vi "Update GUI - Waveform Chart.vi"(6 "Timestamp (optional)":timestamp, 8 "error in (no error)":errorcluster, 9 "Point value":dbl, 10 "GUI Item Name":string, 11 "uService Template in":refnum<class "Father of all uServices.lvclass">) -> (0 "error out":errorcluster, 3 "uService Template out":refnum<class "Father of all uServices.lvclass">)   [LabVIEW 2026, in "TALOS.lvlib" / "Father of all uServices.lvlib" / "Father of all uServices.lvclass"]
doc: "This VI adds a point to the selected Waveform Chart. If not provided externally, this VI will use the time of calling as the timestamp for the point given. \nNote: to properly work, the corresponding indicator in the uService GUI needs to be connected to an empty waveform chart in the Block Diagram of the uService GUI."
uses:
  Father of all uServices.lvclass
  Father of all uServices.lvclass/Father of all uServices.ctl
  Ancestor/Ancestor/Ancestor.lvclass/Ancestor.ctl
  Support VIs/Substitute Error.vi
  Support VIs/Generate Error.vi
  FGV/Error Memory/Get Error Description.vi
  Support VIs/Get PC name.vi
  Ancestor/Ancestor/Read ID.vi
  Support VIs/Get Class Name.vi
  <vilib>/Utility/error.llb/Clear Errors.vi
  FGV/Error Memory/Error Memory Core.vi
  <vilib>/AdvancedString/Delimited String to 1D String Array.vi
  <vilib>/AdvancedString/Delimited String to 1D String Array (string).vi
  Support VIs/Circus Root Path.vi
  FGV/Error Memory/Error Crt Lvl checker.vi
  FGV/Error Memory/Error Memory Core.vi/40c8088d-b597-4017-91af-faa98e00292e.vi
  FGV/Error Memory/Error Memory Core.vi/d4a3ab98-063c-4e44-b43d-fbdcfe6c2be2.vi
  Support VIs/Global Memory.vi
  <vilib>/Utility/LVClass/Get LV Class Name.vi
  Support VIs/Is in Packed Library.vi
  Support VIs/TALOS Root path.vi
  Support VIs/Read CSV worksheet.vi
  Support VIs/Global Constants.vi
  <vilib>/Utility/error.llb/General Error Handler.vi
  Support VIs/Error Log.vi
  Ancestor/Ancestor/Ancestor.lvclass
  <vilib>/Comparison/Equal/Equal Functor/Equal Functor.lvclass
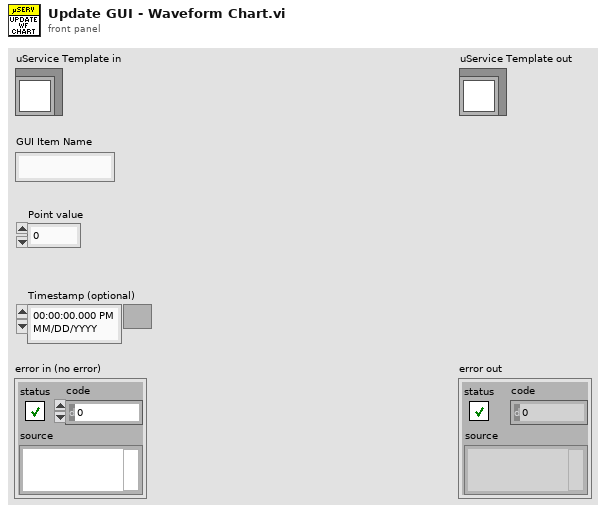
[diagram p1: front panel]
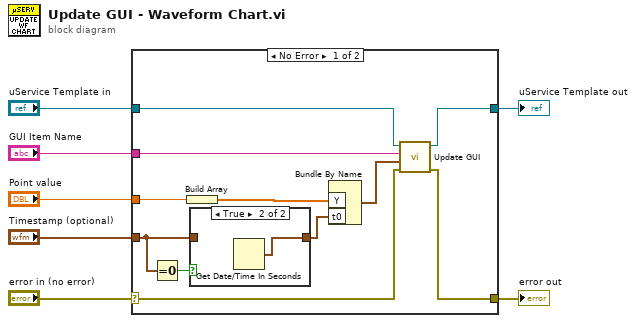
[diagram p0: block diagram]
diagram:
  n1 = case shown="No Error" "error in (no error)" {
    selector: "error in (no error)" -> [w9 w22]
    tunnel: [w8 w22] -> w6
    tunnel: [w12 w21] -> w4
    tunnel: "uService Template in" -> [w13 w21]
    tunnel: "GUI Item Name" -> [w11 _]
    tunnel: "Point value" -> [w18 _]
    tunnel: "Timestamp (optional)" -> [w15 _]
    frame No Error {
      n2 = Equal To 0?(x=w15) -> (x = 0?=w16:bool)
      n3 = Build Array(w18) -> (w17:dbl[])
      n4 = case shown="True" w16 {
        tunnel: w15 -> [w19 _]
        tunnel: [w19 w20] -> w14
        frame False {
        }
        frame True {
          n5 = Get Date/Time In Seconds() -> (seconds since 1Jan1904=w20:timestamp)
        }
      }
      n6 = Bundle By Name("Y"=w17, "t0"=w14) -> (w10:waveform(dbl))  [unwired: 1 in]
      n7 = call "Update GUI.vi"("error in (no error)"=w9, "Data"=w10, "GUI Item Name"=w11, "uService Template in"=w13) -> ("error out"=w8:errorcluster, "uService Template out"=w12:refnum<class "Father of all uServices.lvclass">)  [unwired: 6 in]
    }
    frame Error {
    }
  }
  "error out" <- w6
  "uService Template out" <- w4
